vi "Parse Channels.vi"(4 "tx channel handle array":u32[](array[numeric]), 5 "ScheduledSDI":bool, 6 "rx channel handle array":u32[](array[numeric]), 7 "FIFO Idx Qs":T1, 8 "error in (no error)":errorcluster, 9 "Access":T3, 10 "Section GUID":string, 11 "Device Reference in":T2 format="%.0x") -> (0 "error out":errorcluster, 1 "Section BaseRate":i32, 2 "Section Data":T4[](array[typedef]) {"Labels Settings"."Label" format="%.0o"}, 3 "Device Reference out":T2 format="%.0x")   [LabVIEW 2012, in "AIT 429 Engine.lvlib"]
uses:
  AIT 429 Engine.lvlib
  RT Controls/RT HW Channel.ctl
  RT Controls/RT Label Settings.ctl
  Shared/Controls and Global/Label.ctl
  Shared/Controls and Global/transferPeriod.ctl
  RT Controls/Driver Data.ctl
  RT Controls/RT Word Settings.ctl
  <vilib>/NI Veristand/Custom Device API/Block Data Reference.ctl
  <vilib>/NI Veristand/Custom Device API/Data Reference.ctl
  RT Controls/RT Param Setting.ctl
  Shared/Controls and Global/Start Bit.ctl
  Shared/Controls and Global/Number of Bits.ctl
  Shared/Controls and Global/TransferType.ctl
  <vilib>/NI Veristand/Custom Device API/Data Access Type.ctl
  <vilib>/NI Veristand/Custom Device API/Custom Device Item Ref.ctl
  RT Controls/FIFO Idx Qs.ctl
  <vilib>/NI Veristand/Custom Device Tools/Custom Device Utility Library/NI VeriStand - Search for Item by GUID.vi
  Shared/Controls and Global/Global.vi
  <vilib>/NI Veristand/Custom Device API/Get Item Property (U16).vi
  <vilib>/NI Veristand/Custom Device API/Get Item Property (Double).vi
  <vilib>/NI Veristand/Custom Device Tools/Custom Device Utility Library/Custom Device Utility Library.lvlib
  <vilib>/NI Veristand/Custom Device API/Custom Device API.lvlib
  Shared/ARINC 429 Shared.lvlib
  <vilib>/NI Veristand/Custom Device API/Get Item Property (U32).vi
  <userlib>/ARINC-429/Owl429.lvlib
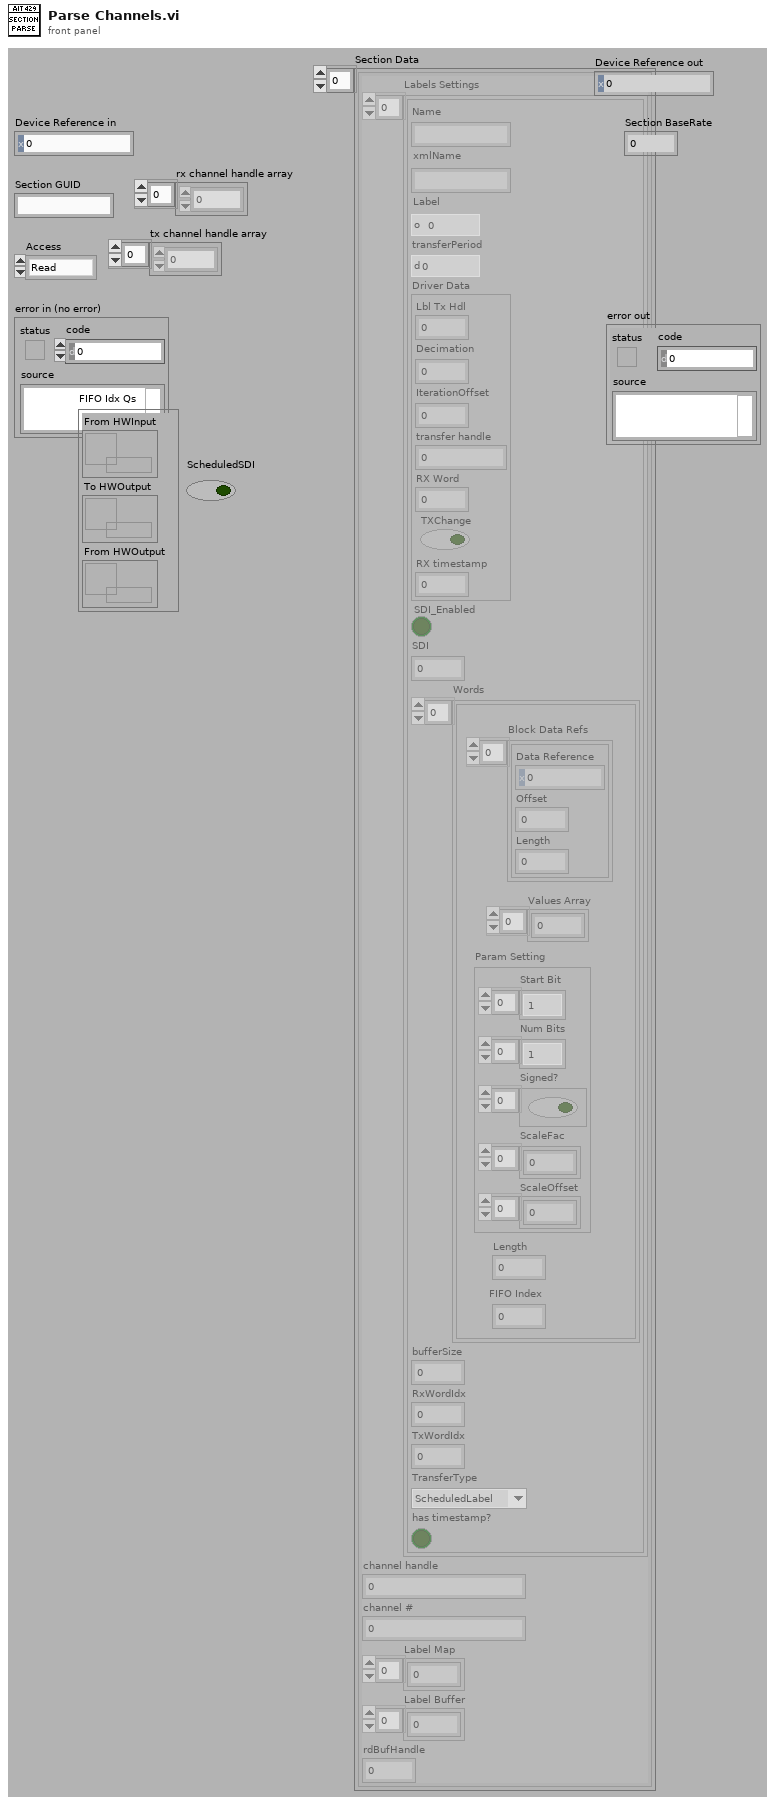
[diagram p1: front panel]
types:
  T1 = typedef "AIT 429 Engine.lvlib/FIFO Idx Qs.ctl" = cluster{"From HWInput":refnum<queue>, "To HWOutput":refnum<queue>, "From HWOutput":refnum<queue>}
  T2 = typedef "Custom Device API.lvlib/Custom Device Item Ref.ctl" = u64
  T3 = typedef "Custom Device API.lvlib/Data Access Type.ctl" = enum16{"Read", "Write"}
  T4 = typedef "AIT 429 Engine.lvlib/RT HW Channel.ctl" = cluster{"Labels Settings":T5[], "channel handle":u32, "channel #":u16, "Label Map":i32[], "Label Buffer":u32[], "rdBufHandle":u32}
  T5 = typedef "AIT 429 Engine.lvlib/RT Label Settings.ctl" = cluster{"Name":string, "xmlName":string, "Label":T6, "transferPeriod":T7, "Driver Data":T8, "SDI_Enabled":bool, "SDI":u8, "Words":T9[], "bufferSize":u32, "RxWordIdx":i32, "TxWordIdx":i32, "TransferType":T15, "has timestamp?":bool}
  T6 = typedef "ARINC 429 Shared.lvlib/Label.ctl" = u8
  T7 = typedef "ARINC 429 Shared.lvlib/transferPeriod.ctl" = u32
  T8 = typedef "AIT 429 Engine.lvlib/Driver Data.ctl" = cluster{"Lbl Tx Hdl":u32, "Decimation":i32, "IterationOffset":i32, "transfer handle":u32, "RX Word":u32, "TXChange":bool, "RX timestamp":dbl}
  T9 = typedef "AIT 429 Engine.lvlib/RT Word Settings.ctl" = cluster{"Block Data Refs":T10[], "Values Array":dbl[], "Length":i32, "FIFO Index":i32, "Param Setting":T12}
  T10 = typedef "Custom Device API.lvlib/Block Data Reference.ctl" = cluster{"Data Reference":T11, "Offset":i32, "Length":i32}
  T11 = typedef "Custom Device API.lvlib/Data Reference.ctl" = i32
  T12 = typedef "AIT 429 Engine.lvlib/RT Param Setting.ctl" = cluster{"Start Bit":T13[], "Num Bits":T14[], "Signed?":bool[], "ScaleFac":dbl[], "ScaleOffset":dbl[]}
  T13 = typedef "ARINC 429 Shared.lvlib/Start Bit.ctl" = i32
  T14 = typedef "ARINC 429 Shared.lvlib/Number of Bits.ctl" = i32
  T15 = typedef "ARINC 429 Shared.lvlib/TransferType.ctl" = enum16{"ScheduledLabel", "Acyclic", "Block", "Strobe"}
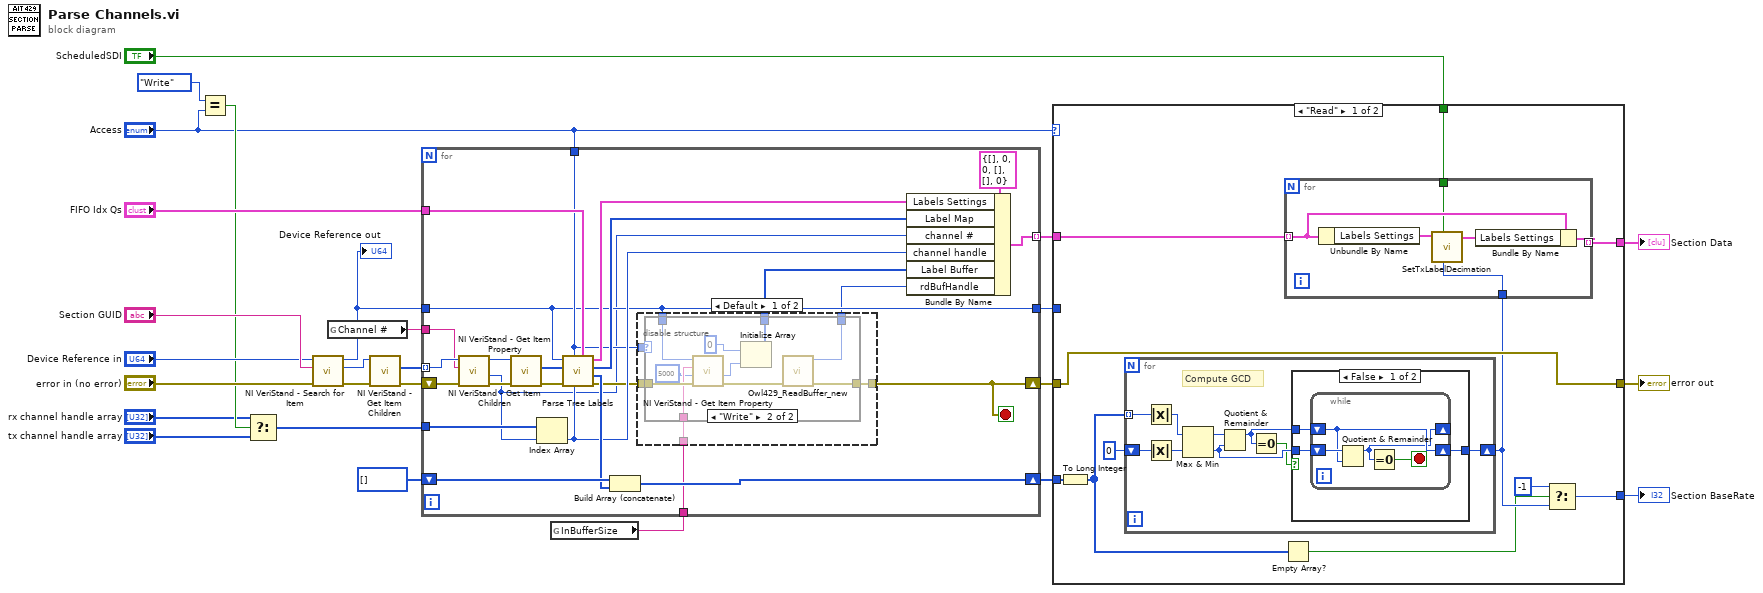
[diagram p0: block diagram]
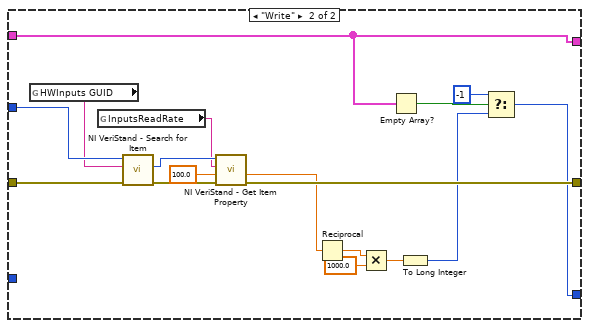
[diagram p3: hidden frame]
diagram:
  n1 = Equal?(x=Data_Access_Type."Write" ("y"), y="Access") -> (x = y?=w11:bool)
  n2 = Select(t="rx channel handle array", s=w11, f="tx channel handle array") -> (s? t:f=w8:u32[])
  n3 = call-poly <vilib>:"NI VeriStand - Search for Item.vi"("error in"="error in (no error)", "Item GUID"="Section GUID", "Section Ref in"="Device Reference in") -> ("error out"=w21:errorcluster, "Item Ref"=w22:T2, "Section Ref out"=w26:T2)  [unwired: 5 in, 1 out]
  "Device Reference out" <- w26
  n4 = global read "Global.vi" "Channel #"() -> (w3:string)
  n5 = call <vilib>:"NI VeriStand - Get Item Children.vi"("error in (no error)"=w21, "Item Ref in"=w22) -> ("error out"=w25:errorcluster, "Child Refs"=w24:T2[])  [unwired: 6 in, 2 out]
  n6 = global read "Global.vi" "InBufferSize"() -> (w2:string)
  n7 = for {
    tunnel: w24 -> [w42] mode=indexing
    tunnel: "Access" -> [w36]
    tunnel: w26 -> [w34]
    tunnel: [w49] -> w16 mode=indexing
    shift-right: [w30] -> w6
    shift-left: w25 -> [w44]
    shift-right: [w45] -> w17
    shift-left: u32[] [] -> [w47]
    tunnel: w8 -> [w39]
    tunnel: "FIFO Idx Qs" -> [w40]
    tunnel: [w34] -> w4
    tunnel: w3 -> [w33]
    tunnel: w2 -> [w32]
    stop <- w30 stop-if-true
    n8 = call-poly <vilib>:"NI VeriStand - Get Item Property.vi"("error in (no error)"=w44, "Property Name"=w33, "Item Ref in"=w42) -> ("error out"=w43:errorcluster, "Value"=w28:u16, "Item Ref out"=w41:T2)  [unwired: 5 in, 1 out]
    n9 = call <vilib>:"NI VeriStand - Get Item Children.vi"("error in (no error)"=w43, "Item Ref in"=w41) -> ("error out"=w48:errorcluster, "Child Refs"=w27:T2[])  [unwired: 6 in, 2 out]
    n10 = Index Array(array=w39, index=w28) -> (element=w38:u32)
    n11 = call "Parse Tree Labels.vi"("FIFO Idx Qs"=w40, "Channel handle in"=w38, "Access"=w36, "error out"=w48, "Label Refs"=w27, "Custom Device Ref"=w34) -> ("error out"=w35:errorcluster, "Transfer Periods"=w46:u32[], "Label Map"=w37:i32[], "Label data"=w50:T5[])  [unwired: 2 in]
    n12 = Build Array (concatenate)(w47, w46) -> (w45:u32[])
    n13 = disable-structure shown="Default" {
      disable-tunnel: w36 -> [w58 _]
      disable-tunnel: w35 -> [w57 w70]
      disable-tunnel: w34 -> [w56 _]
      disable-tunnel: w32 -> [w55 _]
      disable-tunnel: [w54 _] -> w31
      disable-tunnel: [w53 w70] -> w30
      disable-tunnel: [w52 _] -> w29
      frame condition #0 {
        n14 = case shown="\"Write\"" w58 {
          tunnel: w57 -> [w59 w68]
          tunnel: w56 -> [_ w69]
          tunnel: w55 -> [_ w67]
          tunnel: [w59 w61] -> w53
          tunnel: [_ w63] -> w54
          tunnel: [_ w60] -> w52
          frame "Read", Default {
          }
          frame "Write" {
            n15 = call-poly <vilib>:"NI VeriStand - Get Item Property.vi"("error in (no error)"=w68, "Default Value"=u32 5000, "Property Name"=w67, "Item Ref in"=w69) -> ("error out"=w62:errorcluster, "Value"=w65:u32)  [unwired: 4 in, 2 out]
            n16 = Initialize Array(u32 0 ("element"), w65) -> (w63:u32[])
            n17 = call <userlib>:"Owl429_ReadBuffer_new.vi"("error in (no error)"=w62) -> ("error out"=w61:errorcluster, "buffer handle"=w60:u32)  [unwired: 9 in]
          }
        }
      }
      frame condition #1 (active) {
      }
    }
    n18 = Bundle By Name(cluster=T4 {"Labels Settings"=[], "channel handle"=0, "channel #"=0, "Label Map"=[], "Label Buffer"=[], "rdBufHandle"=0} ("HW Channel"), "Labels Settings"=w50, "Label Map"=w37, "channel #"=w28, "channel handle"=w38, "Label Buffer"=w31, "rdBufHandle"=w29) -> (w49:T4)
  }
  n19 = case shown="\"Read\"" "Access" {
    tunnel: w17 -> [w81 _]
    tunnel: w16 -> [w79 w108]
    tunnel: [w75 w105] -> w15
    tunnel: [w78 w108] -> w14
    tunnel: [w77 w115] -> w7
    tunnel: w6 -> [w77 w121]
    tunnel: w4 -> [_ w120]
    tunnel: "ScheduledSDI" -> [w76 _]
    frame "Read" {
      n20 = To Long Integer(number=w81) -> (32bit integer=w74:i32[])
      n21 = for {
        tunnel: w74 -> [w82] mode=indexing
        shift-right: [w84] -> w73
        shift-left: 0 ("gcd(x,y)") -> [w83]
        # "Compute GCD"
        n22 = Absolute Value(x=w82) -> (abs(x)=w89:i32)
        n23 = Absolute Value(x=w83) -> (abs(x)=w90:i32)
        n24 = Max & Min(x=w89, y=w90) -> (max(x,y)=w85:i32, min(x,y)=w87:i32)
        n25 = Quotient & Remainder(x=w85, y=w87) -> (x-y*floor(x/y)=w88:i32)  [unwired: 1 out]
        n26 = Equal To 0?(x=w88) -> (x = 0?=w86:bool)
        n27 = case shown="False" w86 {
          tunnel: [w93 w98] -> w84
          tunnel: w87 -> [w92 w98]
          tunnel: w88 -> [w91 _]
          frame False {
            n28 = while {
              shift-right: [w95] -> w93
              shift-left: w92 -> [w96]
              shift-right: [w94] -> _
              shift-left: w91 -> [w95]
              stop <- w97 stop-if-true
              n29 = Quotient & Remainder(x=w96, y=w95) -> (x-y*floor(x/y)=w94:i32)  [unwired: 1 out]
              n30 = Equal To 0?(x=w94) -> (x = 0?=w97:bool)
            }
          }
          frame True {
          }
        }
      }
      n31 = Empty Array?(array=w74) -> (empty?=w72:bool)
      n32 = for {
        tunnel: w79 -> [w103] mode=indexing
        tunnel: w73 -> [w100]
        tunnel: [w101] -> w78 mode=indexing
        tunnel: w76 -> [w99]
        n33 = Unbundle By Name(w103) -> ("Labels Settings"=w104:T5[])
        n34 = call "SetTxLabelDecimation.vi"("SectionBaseRate"=w100, "ScheduledSDI"=w99, "Labels Settings In"=w104) -> ("Label Settings Out"=w102:T5[])  [unwired: 7 in, 1 out]
        n35 = Bundle By Name(cluster=w103, "Labels Settings"=w102) -> (w101:T4)
      }
      n36 = Select(t=-1, s=w72, f=w73) -> (s? t:f=w75:i32)
    }
    frame "Write" {
      n37 = global read "Global.vi" "HWInputs GUID"() -> (w119:string)
      n38 = global read "Global.vi" "InputsReadRate"() -> (w116:string)
      n39 = call-poly <vilib>:"NI VeriStand - Search for Item.vi"("error in"=w121, "Item GUID"=w119, "Section Ref in"=w120) -> ("error out"=w118:errorcluster, "Item Ref"=w117:T2)  [unwired: 5 in, 2 out]
      n40 = call-poly <vilib>:"NI VeriStand - Get Item Property.vi"("error in (no error)"=w118, "Default Value"=100.0, "Property Name"=w116, "Item Ref in"=w117) -> ("error out"=w115:errorcluster, "Value"=w114:dbl)  [unwired: 4 in, 2 out]
      n41 = Reciprocal(x=w114) -> (1/x=w112:dbl)
      n42 = Multiply(x=w112, y=1000.0) -> (x*y=w110:dbl)
      n43 = Empty Array?(array=w108) -> (empty?=w107:bool)
      n44 = To Long Integer(number=w110) -> (32bit integer=w106:i32)
      n45 = Select(t=-1, s=w107, f=w106) -> (s? t:f=w105:i32)
    }
  }
  "Section Data" <- w14
  "error out" <- w7
  "Section BaseRate" <- w15
